vi "读取配置文件.vi"() -> (0 "簇":T1)   [LabVIEW 2014]
uses:
  <vilib>/Utility/config.llb/Read Key (String).vi
  <vilib>/Utility/config.llb/Read Key (U32).vi
  <vilib>/Utility/config.llb/Read Key (I32).vi
  <vilib>/Utility/config.llb/NI_LVConfig.lvlib
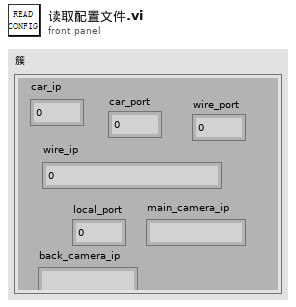
[diagram p1: front panel]
types:
  T1 = cluster{"car_ip":u32, "car_port":i32, "wire_ip":u32, "wire_port":u32, "local_port":u32, "main_camera_ip":string, "back_camera_ip":string}
  T2 = typedef "NI_LVConfig.lvlib/Config Data RefNum.ctl" = refnum<k1>
  T3 = cluster{u32, "value":i32, u32, "value":u32, "value":u32, "value":string, "value":string}
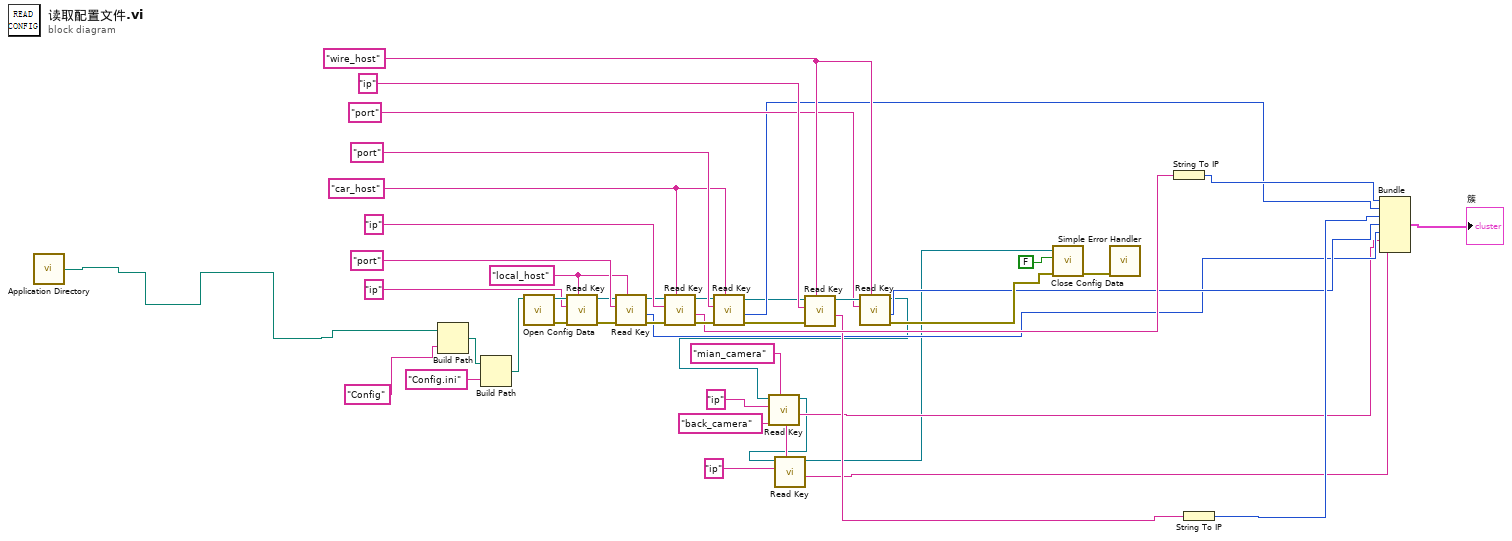
[diagram p0: block diagram]
diagram:
  w21 = "wire_host" ("name or relative path")
  w29 = "car_host" ("name or relative path")
  w33 = "local_host" ("name or relative path")
  n1 = call <vilib>:"Application Directory.vi"() -> ("Application Directory"=w1:path)
  n2 = Build Path(base path=w1, name or relative path="Config") -> (appended path=w45:path)
  n3 = Build Path(base path=w45, name or relative path="Config.ini") -> (appended path=w18:path)
  n4 = call <vilib>:"Open Config Data.vi"("configuration file path"=w18) -> ("error out"=w38:errorcluster, "refnum"=w42:T2)  [unwired: 8 in, 1 out]
  n5 = call-poly <vilib>:"Read Key.vi"("section"=w33, "error in (no error)"=w38, "key"="ip" ("name or relative path"), "refnum"=w42) -> ("error out"=w35:errorcluster, "refnum out"=w36:T2)  [unwired: 2 in, 4 out]
  n6 = call-poly <vilib>:"Read Key.vi"("section"=w33, "error in (no error)"=w35, "key"="port" ("name or relative path"), "refnum"=w36) -> ("error out"=w31:errorcluster, "value"=w13:u32, "refnum out"=w32:T2)  [unwired: 2 in, 3 out]
  n7 = call-poly <vilib>:"Read Key.vi"("section"=w29, "error in (no error)"=w31, "key"="ip" ("name or relative path"), "refnum"=w32) -> ("error out"=w27:errorcluster, "value"=w26:string, "refnum out"=w28:T2)  [unwired: 2 in, 3 out]
  n8 = call-poly <vilib>:"Read Key.vi"("section"=w29, "error in (no error)"=w27, "key"="port" ("name or relative path"), "refnum"=w28) -> ("error out"=w24:errorcluster, "value"=w16:i32, "refnum out"=w7:T2)  [unwired: 2 in, 3 out]
  n9 = call-poly <vilib>:"Read Key.vi"("section"=w21, "error in (no error)"=w24, "key"="ip" ("name or relative path"), "refnum"=w7) -> ("value"=w23:string, "refnum out"=w22:T2)  [unwired: 2 in, 4 out]
  n10 = call-poly <vilib>:"Read Key.vi"("section"=w21, "key"="port" ("name or relative path"), "refnum"=w22) -> ("error out"=w19:errorcluster, "value"=w14:u32, "refnum out"=w4:T2)  [unwired: 3 in, 3 out]
  n11 = call-poly <vilib>:"Read Key.vi"("section"="mian_camera", "key"="ip", "refnum"=w4) -> ("value"=w6:string, "refnum out"=w2:T2)  [unwired: 3 in, 4 out]
  n12 = call-poly <vilib>:"Read Key.vi"("section"="back_camera", "key"="ip", "refnum"=w2) -> ("value"=w5:string, "refnum out"=w3:T2)  [unwired: 3 in, 4 out]
  n13 = call <vilib>:"Close Config Data.vi"("error in (no error)"=w19, "write file if changed (T)"=FALSE ("write configuration file? (T)"), "refnum"=w3) -> ("error out"=w39:errorcluster)  [unwired: 8 out]
  n14 = call <vilib>:"Simple Error Handler.vi"("error in (no error)"=w39) -> ()  [unwired: 1 in, 8 out]
  n15 = String To IP(1:w26) -> (0:w17:u32)
  n16 = String To IP(1:w23) -> (0:w15:u32)
  n17 = Bundle(w17, "value"=w16, w15, "value"=w14, "value"=w13, "value"=w6, "value"=w5) -> (→"簇":T3)  [unwired: 1 in]
